vi "Main.vi"() -> ()   [LabVIEW 2026]
uses:
  <vilib>/Utility/miscctls.llb/LVRowAndColumnTypeDef.ctl
panel:
  out "Com port 3034G":string
  out "error IO":errorcluster
  out "Com port 2260B":string
  in  "device Enum":T1(ring)
  in  "stop":bool
  in  "Tab Control 2":enum32{"編輯指令", "測試項目", "截圖"}(tab)
  in  "Device config Cluster":T2
  in  "Script config Cluster":T3={"Add Button"=FALSE, "Remove Button"=FALSE, "Up Button"=FALSE, "Down Button"=FALSE, "Save Button"=FALSE, "Open Button"=FALSE, "script table"=-1, "快速指令"=enum."常用指令", "data 1-8 Cluster"={"date1"="", "date2"="", "date3"="", "date4"="", "date5"="", "date6"="", "date7"="", "date8"=""}}
  in  "test table":i32(listbox)=2
  in  "Play Button":bool
  in  "Pause Button":bool
  in  "Media Stop Button":bool
  in  "Paste Button":bool=TRUE
  in  "Open Button 4":bool
  out "result table":i32(listbox)
  out "picture array":picture[](array[picture])
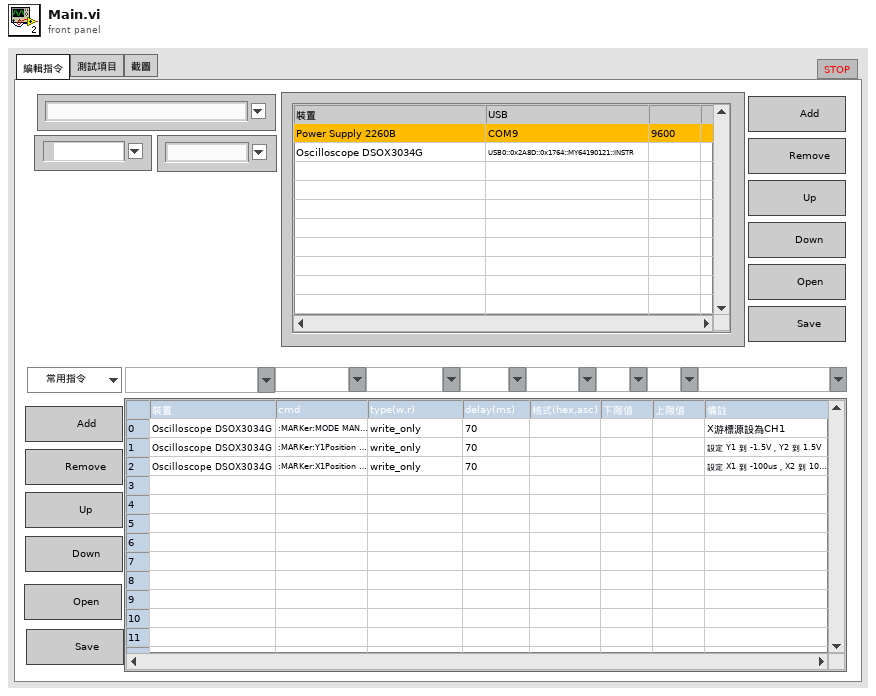
[diagram p1: front panel]
types:
  T1 = enum16{"", "Power Supply 2260B", "Oscilloscope DSOX3034G"}
  T2 = cluster{"Save Button":bool, "Open Button":bool, "Down Button":bool, "Up Button":bool, "Remove Button":bool, "Add Button":bool, "device table":i32, "baud":string, "VISA":refnum<visa-resource-name>, "device":string}
  T3 = cluster{"Add Button":bool, "Remove Button":bool, "Up Button":bool, "Down Button":bool, "Save Button":bool, "Open Button":bool, "script table":i32, "快速指令":enum16{"常用指令", "===Power Supply 2260B===", "問版本號(2260B)", "設定12V", "設定1A", "開啟輸出", "關閉輸出", "電壓量測值?", "電流量測值?", "===Oscilloscope DSOX3034G===", "問版本號(3034G)", "擷取畫面", "CH1開啟", "CH1關閉", "CH1 scal 2V", "CH1 offset -1V", "CH1 cursors XY", "cursor X1X2", "cursor Y1Y2"}, "data 1-8 Cluster":cluster{"date1":string, "date2":string, "date3":string, "date4":string, "date5":string, "date6":string, "date7":string, "date8":string}}
  T4 = typedef "LVRowAndColumnTypeDef.ctl" = cluster{"Row":i32, "Column":i32}
  T5 = cluster{"Com port 2260B":string, "Com port osc":string}
  T6 = cluster{"ItemNames[0]":string, "ItemNames[1]":string, "ItemNames[2]":string, "ItemNames[3]":string, "ItemNames[4]":string, "ItemNames[5]":string, "ItemNames[6]":string, "ItemNames[7]":string}
  T7 = cluster{"date1":string, "date2":string, "date3":string, "date4":string, "date5":string, "date6":string, "date7":string, "date8":string}
  T8 = enum16{"常用指令", "===Power Supply 2260B===", "問版本號(2260B)", "設定12V", "設定1A", "開啟輸出", "關閉輸出", "電壓量測值?", "電流量測值?", "===Oscilloscope DSOX3034G===", "問版本號(3034G)", "擷取畫面", "CH1開啟", "CH1關閉", "CH1 scal 2V", "CH1 offset -1V", "CH1 cursors XY", "cursor X1X2", "cursor Y1Y2"}
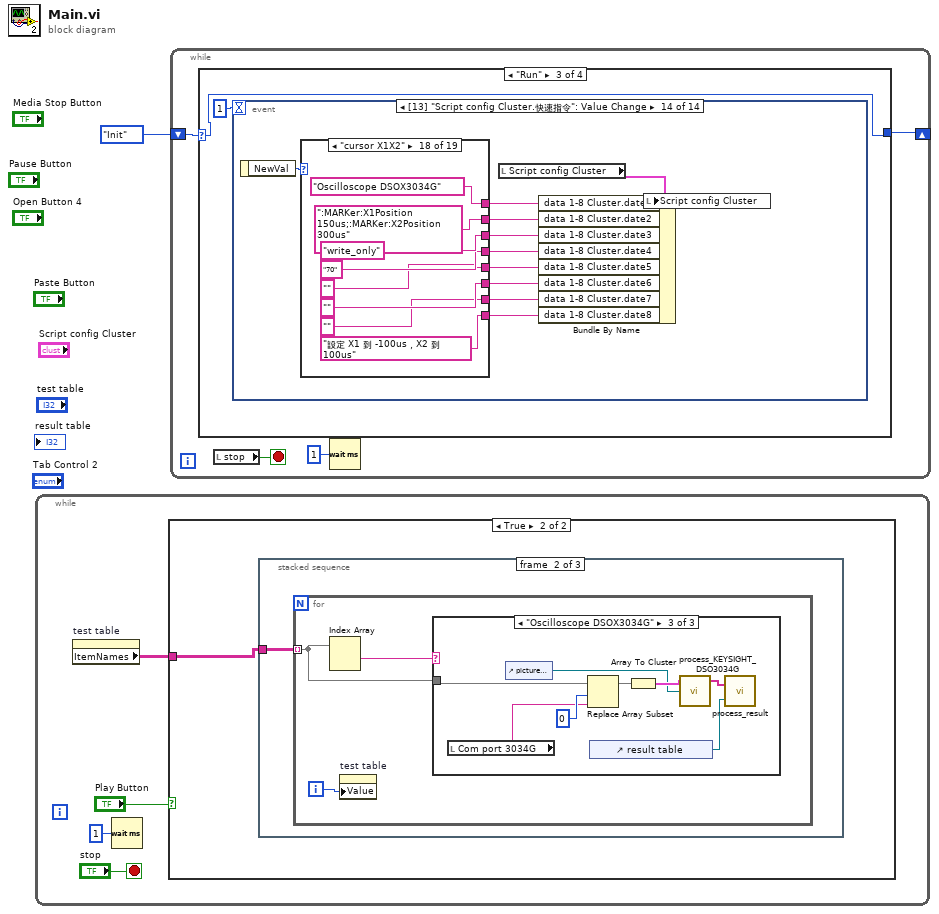
[diagram p0: block diagram]
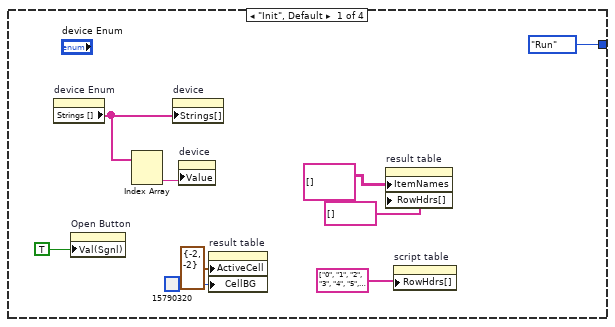
[diagram p2: hidden frame]
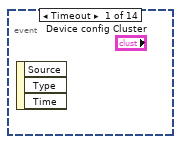
[diagram p4: hidden frame]
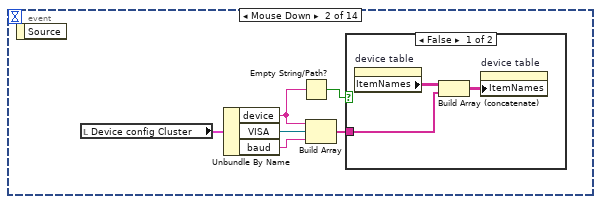
[diagram p5: hidden frame]
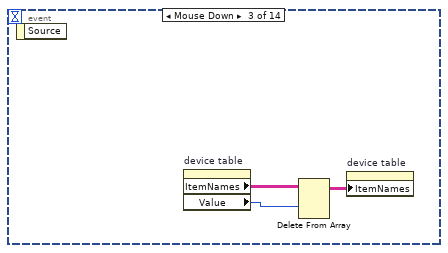
[diagram p7: hidden frame]
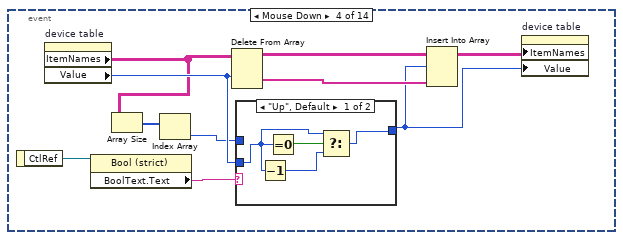
[diagram p8: hidden frame]
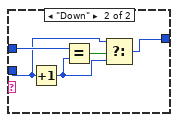
[diagram p9: hidden frame]
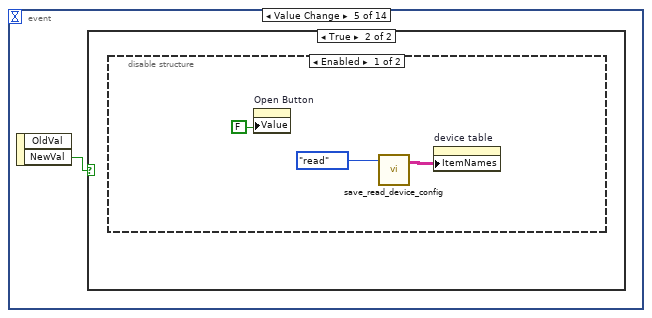
[diagram p10: hidden frame]
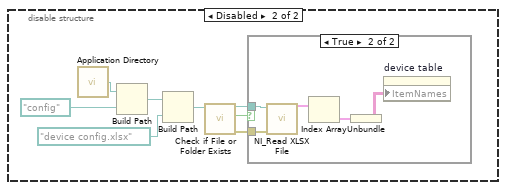
[diagram p12: hidden frame]
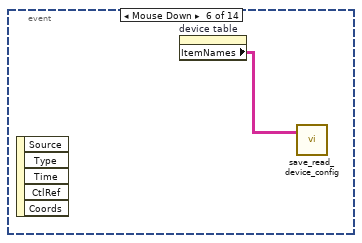
[diagram p14: hidden frame]
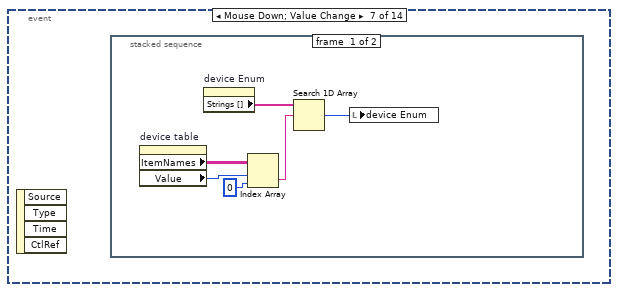
[diagram p15: hidden frame]
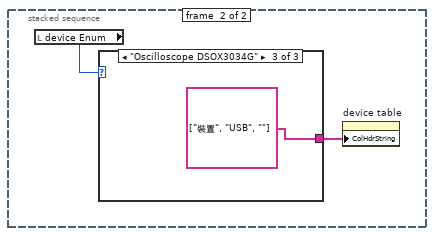
[diagram p16: hidden frame]
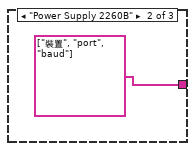
[diagram p18: hidden frame]
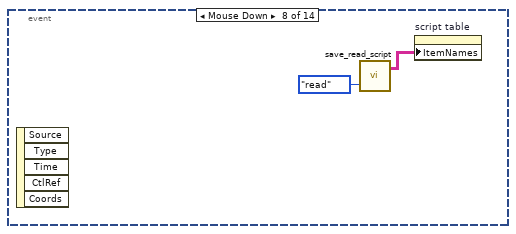
[diagram p19: hidden frame]
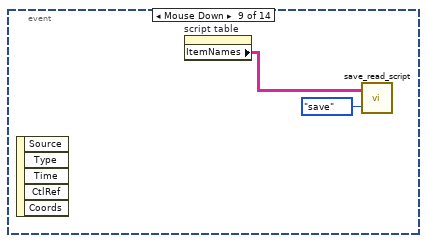
[diagram p20: hidden frame]
diagram:
  n1 = while {
    stop <- "stop" stop-if-true
    n2 = property on="test table" class="MCListbox (strict)"() -> ("ItemNames"=w5:string[][])  [unwired: 2 in, 2 out]
    n3 = Wait (ms)(milliseconds to wait=u32 1) -> ()  [unwired: 1 out]
    n4 = case shown="True" "Play Button" {
      tunnel: w5 -> [_ w6]
      frame False {
      }
      frame True {
        n5 = stacked-sequence {
          tunnel: w6 -> [_ w19 _]
          frame #0 {
            n6 = control-ref of="device table"() -> (w17:refnum<vi>)
            n7 = control-ref of="test table"() -> (w16:refnum<vi>)
            n8 = call "device init.vi"("Enum"=enum16{"none", "open", "close"}."open", "test table"=w16, "device table"=w17) -> ("error IO"=→"error IO":errorcluster, "Cluster"=w14:T5)  [unwired: 1 in]
            n9 = Unbundle By Name(w14) -> ("Com port 2260B"=→"Com port 2260B":string, "Com port osc"=→"Com port 3034G":string)
            n10 = property on="result table" class="MCListbox (strict)"("ItemNames"=string[][] [], "RowHdrs[]"=string[] [] ("Row Header Strings[]"), "ActiveCell"=T4 {"Row"=-2, "Column"=-2} ("Active Cell:Active Cell"), "CellBG"=u32 15790320 ("Active Cell:Cell Background Color")) -> ()  [unwired: 2 in, 2 out]
            "picture array" <- picture[] [] ("picture array")
          }
          frame #1 {
            n11 = for {
              tunnel: w19 -> [w20] mode=indexing
              i -> [w21]
              n12 = Index Array(array=w20) -> (element #1=w22:string)  [unwired: 2 in, 1 out]
              n13 = property on="test table" class="MCListbox (strict)"("Value"=w21) -> ()  [unwired: 2 in, 2 out]
              n14 = case shown="\"Oscilloscope DSOX3034G\"" w22 {
                tunnel: w20 -> [_ w29 w34]
                frame "False", Default {
                }
                frame "Power Supply 2260B" {
                  n15 = local read "Com port 2260B"() -> (w23:string)
                  n16 = Replace Array Subset(array=w29, new element=w23, index=0) -> (w27:string[])
                  n17 = control-ref of="result table"() -> (w24:refnum<vi>)
                  n18 = Array To Cluster(array=w27) -> (cluster=w26:T6)
                  n19 = call "process_KEITHLEY_2260B.vi"("Cluster"=w26) -> ("2260B_output"=w25:string[])  [unwired: 1 in, 1 out]
                  n20 = call "process_result.vi"("reference 2"=w24, "reuslt cmd"=w25) -> ()  [unwired: 2 in]
                }
                frame "Oscilloscope DSOX3034G" {
                  n21 = local read "Com port 3034G"() -> (w33:string)
                  n22 = control-ref of="picture array"() -> (w30:refnum<vi>)
                  n23 = Replace Array Subset(array=w34, new element=w33, index=0) -> (w37:string[])
                  n24 = control-ref of="result table"() -> (w36:refnum<vi>)
                  n25 = Array To Cluster(array=w37) -> (cluster=w32:T6)
                  n26 = call "process_KEYSIGHT_DSO3034G.vi"("Array 2"=w30, "Cluster"=w32) -> ("DSO3034G_output"=w31:string[])  [unwired: 2 in, 1 out]
                  n27 = call "process_result.vi"("reference 2"=w36, "reuslt cmd"=w31) -> ()  [unwired: 2 in]
                }
              }
            }
          }
          frame #2 {
            n28 = control-ref of="device table"() -> (w41:refnum<vi>)
            n29 = control-ref of="test table"() -> (w40:refnum<vi>)
            n30 = local write "Play Button"(FALSE ("Play Button")) -> ()
            n31 = call "device init.vi"("Enum"=enum16{"none", "open", "close"}."close", "test table"=w40, "device table"=w41) -> ()  [unwired: 1 in, 2 out]
          }
        }
      }
    }
  }
  n32 = while {
    shift-right: [w42] -> _
    shift-left: enum16{"Init", "Idle", "Run", "Stop"}."Init" -> [w43]
    stop <- w45 stop-if-true
    n33 = case shown="\"Run\"" w43 {
      selector: w43 -> [_ _ w55 _]
      tunnel: [enum16{"Init", "Idle", "Run", "Stop"}."Run" _ w55 _] -> w42
      frame "Init", Default {
        n34 = property on="device Enum" class="Enum (strict)"() -> ("Strings []"=w52:string[])  [unwired: 2 in, 2 out]
        n35 = property on="Open Button" class="Bool (strict)"("Val(Sgnl)"=TRUE ("Value")) -> ()  [unwired: 2 in, 2 out]
        n36 = Index Array(array=w52) -> (element #2=w53:string)  [unwired: 2 in, 1 out]
        n37 = property on="device" class="CmbBox"("Strings[]"=w52) -> ()  [unwired: 2 in, 2 out]
        n38 = property on="device" class="CmbBox"("Value"=w53) -> ()  [unwired: 2 in, 2 out]
        n39 = property on="result table" class="MCListbox (strict)"("ActiveCell"=T4 {"Row"=-2, "Column"=-2} ("Active Cell:Active Cell"), "CellBG"=u32 15790320 ("Active Cell:Cell Background Color")) -> ()  [unwired: 2 in, 2 out]
        n40 = property on="result table" class="MCListbox (strict)"("ItemNames"=string[][] [], "RowHdrs[]"=string[] [] ("Row Header Strings[]")) -> ()  [unwired: 2 in, 2 out]
        n41 = property on="script table" class="MCListbox (strict)"("RowHdrs[]"=string[] ["0", "1", "2", "3", "4", "5", "6", "7", "8", "9", "10", "11", "12", "13", "14", "15", "16", "17", "18", "19", "20", "21", "22", "23", "24", "25", "26", "27", "28", "29", "30", "31", "32", "33", "34", "35", "36", "37", "38", "39", "40", "41", "42", "43", "44", "45", "46", "47", "48", "49", "50", "51", "52", "53", "54", "55", "56", "57", "58", "59", "60", "61", "62", "63", "64", "65", "66", "67", "68", "69", "70", "71", "72", "73", "74", "75", "76", "77", "78", "79", "80", "81", "82", "83", "84", "85", "86", "87", "88", "89", "90", "91", "92", "93", "94", "95", "96", "97", "98", "99"] ("Array")) -> ()  [unwired: 2 in, 2 out]
      }
      frame "Idle" {
      }
      frame "Run" {
        n42 = event shown="[13] \"Script config Cluster.快速指令\": Value Change" {
          selector: _ -> [_ _ _ _ _ _ _ _ _ _ _ _ _ _]
          dyn-events: _ -> [_ _ _ _ _ _ _ _ _ _ _ _ _ _]
          timeout: 1 -> [_ _ _ _ _ _ _ _ _ _ _ _ _ _]
          event Timeout {
            n43 = event-data() -> ()  [unwired: 1 in, 3 out]
          }
          event "Device config Cluster.Add Button": Mouse Down {
            n44 = event-data() -> ()  [unwired: 1 in, 1 out]
            n45 = local read "Device config Cluster"() -> (w62:T2)
            n46 = Unbundle By Name(w62) -> ("device"=w58:string, "VISA"=w61:refnum<visa-resource-name>, "baud"=w60:string)
            n47 = Empty String/Path?(string/path=w58) -> (empty?=w57:bool)
            n48 = Build Array(w58, w61, w60) -> (w59:string[])
            n49 = case shown="False" w57 {
              tunnel: w59 -> [w63 _]
              frame False {
                n50 = property on="device table" class="MCListbox (strict)"() -> ("ItemNames"=w64:string[][])  [unwired: 2 in, 2 out]
                n51 = Build Array (concatenate)(w64, w63) -> (w65:string[][])
                n52 = property on="device table" class="MCListbox (strict)"("ItemNames"=w65) -> ()  [unwired: 2 in, 2 out]
              }
              frame True {
              }
            }
          }
          event "Device config Cluster.Remove Button": Mouse Down {
            n53 = event-data() -> ()  [unwired: 1 in, 1 out]
            n54 = property on="device table" class="MCListbox (strict)"() -> ("ItemNames"=w67:string[][], "Value"=w66:i32)  [unwired: 2 in, 2 out]
            n55 = Delete From Array(array=w67, index (row)=w66) -> (array with subset deleted=w68:string[][])  [unwired: 2 in, 1 out]
            n56 = property on="device table" class="MCListbox (strict)"("ItemNames"=w68) -> ()  [unwired: 2 in, 2 out]
          }
          event "Device config Cluster.Down Button", "Device config Cluster.Up Button": Mouse Down {
            n57 = event-data() -> ("CtlRef"=w75:refnum<vi>)  [unwired: 1 in]
            n58 = property on="device table" class="MCListbox (strict)"() -> ("ItemNames"=w71:string[][], "Value"=w73:i32)  [unwired: 2 in, 2 out]
            n59 = property class="Bool (strict)"(reference=w75) -> ("BoolText.Text"=w74:string)  [unwired: 1 in, 2 out]
            n60 = Array Size(array=w71) -> (size(s)=w70:i32[])
            n61 = Index Array(array=w70) -> (element=w69:i32)  [unwired: 1 in]
            n62 = Delete From Array(array=w71, index (row)=w73) -> (deleted portion=w76:string[], array with subset deleted=w78:string[][])  [unwired: 2 in]
            n63 = case shown="\"Up\", Default" w74 {
              tunnel: w73 -> [w80 w83]
              tunnel: [w79 w84] -> w72
              tunnel: w69 -> [_ w86]
              frame "Up", Default {
                n64 = Decrement(x=w80) -> (x-1=w81:i32)
                n65 = Equal To 0?(x=w80) -> (x = 0?=w82:bool)
                n66 = Select(t=w80, s=w82, f=w81) -> (s? t:f=w79:i32)
              }
              frame "Down" {
                n67 = Increment(x=w83) -> (x+1=w85:i32)
                n68 = Equal?(x=w86, y=w85) -> (x = y?=w87:bool)
                n69 = Select(t=w83, s=w87, f=w85) -> (s? t:f=w84:i32)
              }
            }
            n70 = Insert Into Array(array=w78, index (row)=w72, new element=w76) -> (w77:string[][])  [unwired: 1 in]
            n71 = property on="device table" class="MCListbox (strict)"("ItemNames"=w77, "Value"=w72) -> ()  [unwired: 2 in, 2 out]
          }
          event "Device config Cluster.Open Button": Value Change {
            n72 = event-data() -> ("NewVal"=w88:bool)  [unwired: 1 in, 1 out]
            n73 = case shown="True" w88 {
              frame False {
              }
              frame True {
                n74 = disable-structure shown="Enabled" {
                  frame Enabled {
                    n75 = property on="Open Button" class="Bool (strict)"("Value"=FALSE) -> ()  [unwired: 2 in, 2 out]
                    n76 = call "save_read_device_config.vi"("w-r"=enum16{"save", "read"}."read") -> ("output table"=w90:string[][])  [unwired: 1 in, 1 out]
                    n77 = property on="device table" class="MCListbox (strict)"("ItemNames"=w90) -> ()  [unwired: 2 in, 2 out]
                  }
                  frame Disabled {
                    n78 = call <vilib>:"Application Directory.vi"() -> ("Application Directory"=w94:path)
                    n79 = Build Path(base path=w94, name or relative path=path "config") -> (appended path=w95:path)
                    n80 = Build Path(base path=w95, name or relative path=path "device config.xlsx") -> (appended path=w96:path)
                    n81 = call <vilib>:"Check if File or Folder Exists.vi"("path"=w96) -> ("error out"=w99:errorcluster, "file or folder exists?"=w97:bool, "dup path"=w98:path)  [unwired: 8 in]
                    n82 = case shown="True" w97 {
                      tunnel: w98 -> [_ w104]
                      tunnel: w99 -> [_ w101]
                      frame False {
                      }
                      frame True {
                        n83 = call "NI_Read XLSX File.vi"("error in"=w101, "XLSX File"=w104) -> ("Sheet Data"=w103:cluster{"Array":string[][]}[])  [unwired: 7 in, 2 out]
                        n84 = Index Array(array=w103) -> (element=w102:cluster{"Array":string[][]})  [unwired: 1 in]
                        n85 = Unbundle(w102) -> ("Array"=w100:string[][])
                        n86 = property on="device table" class="MCListbox (strict)"("ItemNames"=w100) -> ()  [unwired: 2 in, 2 out]
                      }
                    }
                  }
                }
              }
            }
          }
          event "Device config Cluster.Save Button": Mouse Down {
            n87 = event-data() -> ()  [unwired: 1 in, 5 out]
            n88 = property on="device table" class="MCListbox (strict)"() -> ("ItemNames"=w105:string[][])  [unwired: 2 in, 2 out]
            n89 = call "save_read_device_config.vi"("intput table"=w105) -> ()  [unwired: 1 in, 2 out]
          }
          event "Device config Cluster.device table": Mouse Down; "Device config Cluster.device table": Value Change {
            n90 = event-data() -> ()  [unwired: 1 in, 4 out]
            n91 = stacked-sequence {
              frame #0 {
                n92 = property on="device table" class="MCListbox (strict)"() -> ("ItemNames"=w111:string[][], "Value"=w109:i32)  [unwired: 2 in, 2 out]
                n93 = property on="device Enum" class="Enum (strict)"() -> ("Strings []"=w108:string[])  [unwired: 2 in, 2 out]
                n94 = Index Array(array=w111, index (row)=w109, index (col)=0 ("index (row)")) -> (element=w107:string)
                n95 = Search 1D Array(1D array=w108, element=w107) -> (index of element=w106:i32)  [unwired: 1 in]
                n96 = local write "device Enum"(w106) -> ()
              }
              frame #1 {
                n97 = local read "device Enum"() -> (w113:T1)
                n98 = case shown="\"Oscilloscope DSOX3034G\"" w113 {
                  tunnel: [_ string[] ["裝置", "port", "baud"] string[] ["裝置", "USB", ""]] -> w112
                  frame "", Default {
                  }
                  frame "Power Supply 2260B" {
                  }
                  frame "Oscilloscope DSOX3034G" {
                  }
                }
                n99 = property on="device table" class="MCListbox (strict)"("ColHdrString"=w112) -> ()  [unwired: 2 in, 2 out]
              }
            }
          }
          event "Script config Cluster.Open Button": Mouse Down {
            n100 = event-data() -> ()  [unwired: 1 in, 5 out]
            n101 = call "save_read_script.vi"("w-r"=enum16{"save", "read"}."read") -> ("output table"=w116:string[][])  [unwired: 1 in, 1 out]
            n102 = property on="script table" class="MCListbox (strict)"("ItemNames"=w116) -> ()  [unwired: 2 in, 2 out]
          }
          event "Script config Cluster.Save Button": Mouse Down {
            n103 = event-data() -> ()  [unwired: 1 in, 5 out]
            n104 = property on="script table" class="MCListbox (strict)"() -> ("ItemNames"=w118:string[][])  [unwired: 2 in, 2 out]
            n105 = call "save_read_script.vi"("w-r"=enum16{"save", "read"}."save", "intput table"=w118) -> ()  [unwired: 2 out]
          }
          event "Script config Cluster.Add Button": Mouse Down {
            n106 = event-data() -> ()  [unwired: 1 in, 5 out]
            n107 = local read "Script config Cluster"() -> (w129:T3)
            n108 = Unbundle By Name(w129) -> ("data 1-8 Cluster"=w128:T7)
            n109 = Unbundle(w128) -> ("date1"=w127:string, "date2"=w126:string, "date3"=w125:string, "date4"=w124:string, "date5"=w123:string, "date6"=w122:string, "date7"=w121:string, "date8"=w120:string)
            n110 = Build Array(w127, w126, w125, w124, w123, w122, w121, w120) -> (w132:string[])
            n111 = Empty String/Path?(string/path=w132) -> (empty?=w131:bool[])
            n112 = And Array Elements(Boolean array=w131) -> (logical AND=w130:bool)
            n113 = case shown="False" w130 {
              tunnel: w132 -> [w133 _]
              frame False {
                n114 = property on="script table" class="MCListbox (strict)"() -> ("ItemNames"=w135:string[][])  [unwired: 2 in, 2 out]
                n115 = Build Array (concatenate)(w135, w133) -> (w134:string[][])
                n116 = property on="script table" class="MCListbox (strict)"("ItemNames"=w134) -> ()  [unwired: 2 in, 2 out]
              }
              frame True {
              }
            }
          }
          event "Script config Cluster.Remove Button": Mouse Down {
            n117 = event-data() -> ()  [unwired: 1 in, 5 out]
            n118 = property on="script table" class="MCListbox (strict)"() -> ("ItemNames"=w137:string[][], "Value"=w136:i32)  [unwired: 2 in, 2 out]
            n119 = Delete From Array(array=w137, index (row)=w136) -> (array with subset deleted=w138:string[][])  [unwired: 2 in, 1 out]
            n120 = property on="script table" class="MCListbox (strict)"("ItemNames"=w138) -> ()  [unwired: 2 in, 2 out]
          }
          event "Script config Cluster.Up Button", "Script config Cluster.Down Button": Mouse Down {
            n121 = event-data() -> ("CtlRef"=w139:refnum<vi>)  [unwired: 1 in]
            n122 = property on="script table" class="MCListbox (strict)"() -> ("ItemNames"=w142:string[][], "Value"=w144:i32)  [unwired: 2 in, 2 out]
            n123 = property class="Bool (strict)"(reference=w139) -> ("BoolText.Text"=w145:string)  [unwired: 1 in, 2 out]
            n124 = Array Size(array=w142) -> (size(s)=w141:i32[])
            n125 = Index Array(array=w141) -> (element=w140:i32)  [unwired: 1 in]
            n126 = Delete From Array(array=w142, index (row)=w144) -> (deleted portion=w146:string[], array with subset deleted=w148:string[][])  [unwired: 2 in]
            n127 = case shown="\"Up\", Default" w145 {
              tunnel: w144 -> [w150 w153]
              tunnel: [w149 w154] -> w143
              tunnel: w140 -> [_ w156]
              frame "Up", Default {
                n128 = Decrement(x=w150) -> (x-1=w151:i32)
                n129 = Equal To 0?(x=w150) -> (x = 0?=w152:bool)
                n130 = Select(t=w150, s=w152, f=w151) -> (s? t:f=w149:i32)
              }
              frame "Down" {
                n131 = Increment(x=w153) -> (x+1=w155:i32)
                n132 = Equal?(x=w156, y=w155) -> (x = y?=w157:bool)
                n133 = Select(t=w153, s=w157, f=w155) -> (s? t:f=w154:i32)
              }
            }
            n134 = Insert Into Array(array=w148, index (row)=w143, new element=w146) -> (w147:string[][])  [unwired: 1 in]
            n135 = property on="script table" class="MCListbox (strict)"("ItemNames"=w147, "Value"=w143) -> ()  [unwired: 2 in, 2 out]
          }
          event "Open Button 4": Mouse Down {
            n136 = event-data() -> ()  [unwired: 1 in, 6 out]
            n137 = call "save_read_script.vi"("w-r"=enum16{"save", "read"}."read") -> ("output table"=w159:string[][])  [unwired: 1 in, 1 out]
            n138 = property on="test table" class="MCListbox (strict)"("ItemNames"=w159) -> ()  [unwired: 2 in, 2 out]
          }
          event "Script config Cluster.快速指令": Value Change {
            n139 = event-data() -> ("NewVal"=w170:T8)  [unwired: 1 in]
            n140 = case shown="\"cursor X1X2\"" w170 {
              tunnel: [_ _ "Power Supply 2260B" "Power Supply 2260B" "Power Supply 2260B" "Power Supply 2260B" "Power Supply 2260B" "Power Supply 2260B" "Power Supply 2260B" _ "Oscilloscope DSOX3034G" "Oscilloscope DSOX3034G" "Oscilloscope DSOX3034G" "Oscilloscope DSOX3034G" "Oscilloscope DSOX3034G" "Oscilloscope DSOX3034G" "Oscilloscope DSOX3034G" "Oscilloscope DSOX3034G" "Oscilloscope DSOX3034G"] -> w167
              tunnel: [_ _ "*IDN?" "SOUR:VOLT 12.0" "SOUR:CURR 1.0" "OUTP 1" "OUTP 0" "MEAS:VOLT?" "MEAS:CURR?" _ "*IDN?" ":DISPlay:DATA? PNG, COLOR" ":CHAN1:DISP ON;" ":CHAN1:DISP OFF;" ":CHAN1:SCAL 2.000;\t" ":CHAN1:OFFS -1;" ":MARKer:MODE MANual;:MARKer:X1Y1source CHANnel1" ":MARKer:X1Position 150us;:MARKer:X2Position 300us" ":MARKer:Y1Position -1.5;:MARKer:Y2Position 1.5"] -> w166
              tunnel: [_ _ "write_only" "write_only" "write_only" "write_only" "write_only" "write_and_read" "write_and_read" _ "write_and_read" "scope" "write_only" "write_only" "write_only" "write_only" "write_only" "write_only" "write_only"] -> w165
              tunnel: [_ _ "70" "70" "70" "70" "70" "70" "70" _ "70" "" "70" "70" "70" "70" "70" "70" "70"] -> w164
              tunnel: [_ _ "asc,search" "" "asc,search" "asc,search" "asc,search" "float" "float" _ "asc,search" "" "" "" "" "" "" "" _] -> w163
              tunnel: [_ _ "2260B" "" "2260B" "2260B" "2260B" "15" "5" _ "3034G" "" "" "" "" "" "" "" _] -> w162
              tunnel: [_ _ "2260B" "" "2260B" "2260B" "2260B" "10" "1" _ "3034G" "" "" "" "" "" "" "" _] -> w161
              tunnel: [_ _ "設備型號" "設定輸出12V" "設定輸出1A" "開啟輸出" "設備型號" "電壓量測值" "電流量測值" _ "設備型號" "擷取畫面" "channel open" "channel open" "CH1 scale 2V" "CH1 offset -1V" "X游標源設為CH1" "設定 X1 到 -100us，X2 到 100us" "設定 Y1 到 -1.5V，Y2 到 1.5V"] -> w160
              frame "常用指令", Default {
              }
              frame "===Power Supply 2260B===" {
              }
              frame "問版本號(2260B)" {
              }
              frame "設定12V" {
              }
              frame "設定1A" {
              }
              frame "開啟輸出" {
              }
              frame "關閉輸出" {
              }
              frame "電壓量測值?" {
              }
              frame "電流量測值?" {
              }
              frame "===Oscilloscope DSOX3034G===" {
              }
              frame "問版本號(3034G)" {
              }
              frame "擷取畫面" {
              }
              frame "CH1開啟" {
              }
              frame "CH1關閉" {
              }
              frame "CH1 scal 2V" {
              }
              frame "CH1 offset -1V" {
              }
              frame "CH1 cursors XY" {
              }
              frame "cursor X1X2" {
              }
              frame "cursor Y1Y2" {
              }
            }
            n141 = local read "Script config Cluster"() -> (w169:T3)
            n142 = Bundle By Name(cluster=w169, "data 1-8 Cluster.date1"=w167, "data 1-8 Cluster.date2"=w166, "data 1-8 Cluster.date3"=w165, "data 1-8 Cluster.date4"=w164, "data 1-8 Cluster.date5"=w163, "data 1-8 Cluster.date6"=w161, "data 1-8 Cluster.date7"=w162, "data 1-8 Cluster.date8"=w160) -> (w168:T3)
            n143 = local write "Script config Cluster"(w168) -> ()
          }
        }
      }
      frame "Stop" {
      }
    }
    n144 = local read "stop"() -> (w45:bool)
    n145 = Wait (ms)(milliseconds to wait=u32 1) -> ()  [unwired: 1 out]
  }
